vi "STM Multi-Client - Command Server.vi"() -> ()   [LabVIEW 2016]
uses:
  <vilib>/NI/STM/Connection Manager/TCP/TCP Connection Method.ctl
  <vilib>/NI/STM/SubVIs/MetaDataElement.ctl
  <vilib>/Platform/TimedLoop/XDataNode/timing_clust.ctl
  <vilib>/Platform/TimedLoop/XDataNode/nitl_modes.ctl
  <vilib>/Platform/TimedLoop/XDataNode/wakeup.ctl
  <vilib>/NI/STM/TCP/Write Meta Data (TCP Ref).vi
  <vilib>/NI/STM/TCP/Read Message (TCP).vi
  <vilib>/NI/STM/TCP/Write Message (TCP).vi
  <vilib>/NI/STM/TCP/Write Meta Data (TCP Clst).vi
  <vilib>/Platform/TimedLoop/XDataNode/XDataNode.xnode
  <vilib>/Platform/TimedLoop/XDataNode/XDNodeRunTimeDep.lvlib
  <vilib>/NI/STM/NI STM.lvlib
panel:
  in  "Stop non-critical loops":bool
  out "error out":errorcluster
  out "Number of \nConnections":i32
  # "Overview: Demonstrate the use of the STM library to implement a Single Server Multi Client application design. \nRequirements: LabVIEW Full Development System, STM Library version 3.x or later\nInstructions: \n1. Run the STM Multi-Client - Server VI\n2. Set the Target IP Address in the STM Multi-Client - Client VI to match the IP address of the server\n3. Run the STM Multi-Client - Client VI\n4. Change the Channel to choose between four different waveform"
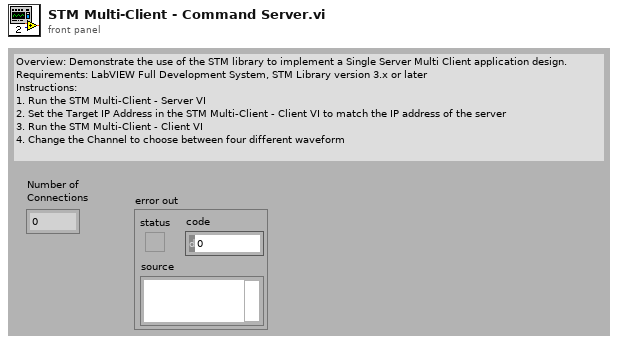
[diagram p1: front panel]
types:
  T1 = typedef "NI STM.lvlib/TCP Connection Method.ctl" = enum16{"Initialize", "Add Connection", "Set Properties", "Get Connection(s)", "Remove Connection", "Remove All Connections", "Get Connection Count"}
  T2 = typedef "NI STM.lvlib/MetaDataElement.ctl" = string
  T3 = typedef "FIFOs (STM Multi-Client).ctl" = cluster{"Data FIFO":refnum<queue>, "Stop FIFO":refnum<queue>}
  T4 = typedef "XDNodeRunTimeDep.lvlib/timing_clust.ctl" = cluster{"Expected End [f-1]":u64, "Actual End [f-1]":u64, "Finished Late? [f-1]":bool, "Expected End [i-1]":u64, "Actual End [i-1]":u64, "Finished Late? [i-1]":bool, "Expected Start [i]":u64, "Actual Start [i]":u64, "Expected Start [f]":u64, "Actual Start [f]":u64, "Source Name":string, "Structure Name":string, "Period":i64, "Deadline":i64, "Offset":i64, "Start":i64, "Priority":i32, "Timeout":i32, "Mode":T5, "Wakeup Reason":T6, "Error":errorcluster, "Source Type":string, "Secondary Source Type":string, "Global End Time":u64, "Global Start Time":u64, "Frame Duration":u64, "Iteration Duration":u64, "Assigned CPU":i32, "I/O Scan Engine Mode":u32}
  T5 = typedef "XDNodeRunTimeDep.lvlib/nitl_modes.ctl" = enum32{"No Change", "Process missed periods, maintain original phase", "Discard missed periods, maintain original phase", "Process missed periods, ignore original phase", "Discard missed periods, ignore original phase"}
  T6 = typedef "XDNodeRunTimeDep.lvlib/wakeup.ctl" = enum32{"Normal", "Aborted", "Asynchronous wakeup", "Timing source error", "Timed loop error", "Timeout"}
  T7 = typedef "NI STM.lvlib/TCP Connection Info.ctl" = cluster{"connection ID":refnum<k5>, "meta data":T2[]}
  T8 = typedef "NI STM.lvlib/TCP Connection Properties.ctl" = cluster{"Name":string, "Address":string, "Custom":string}
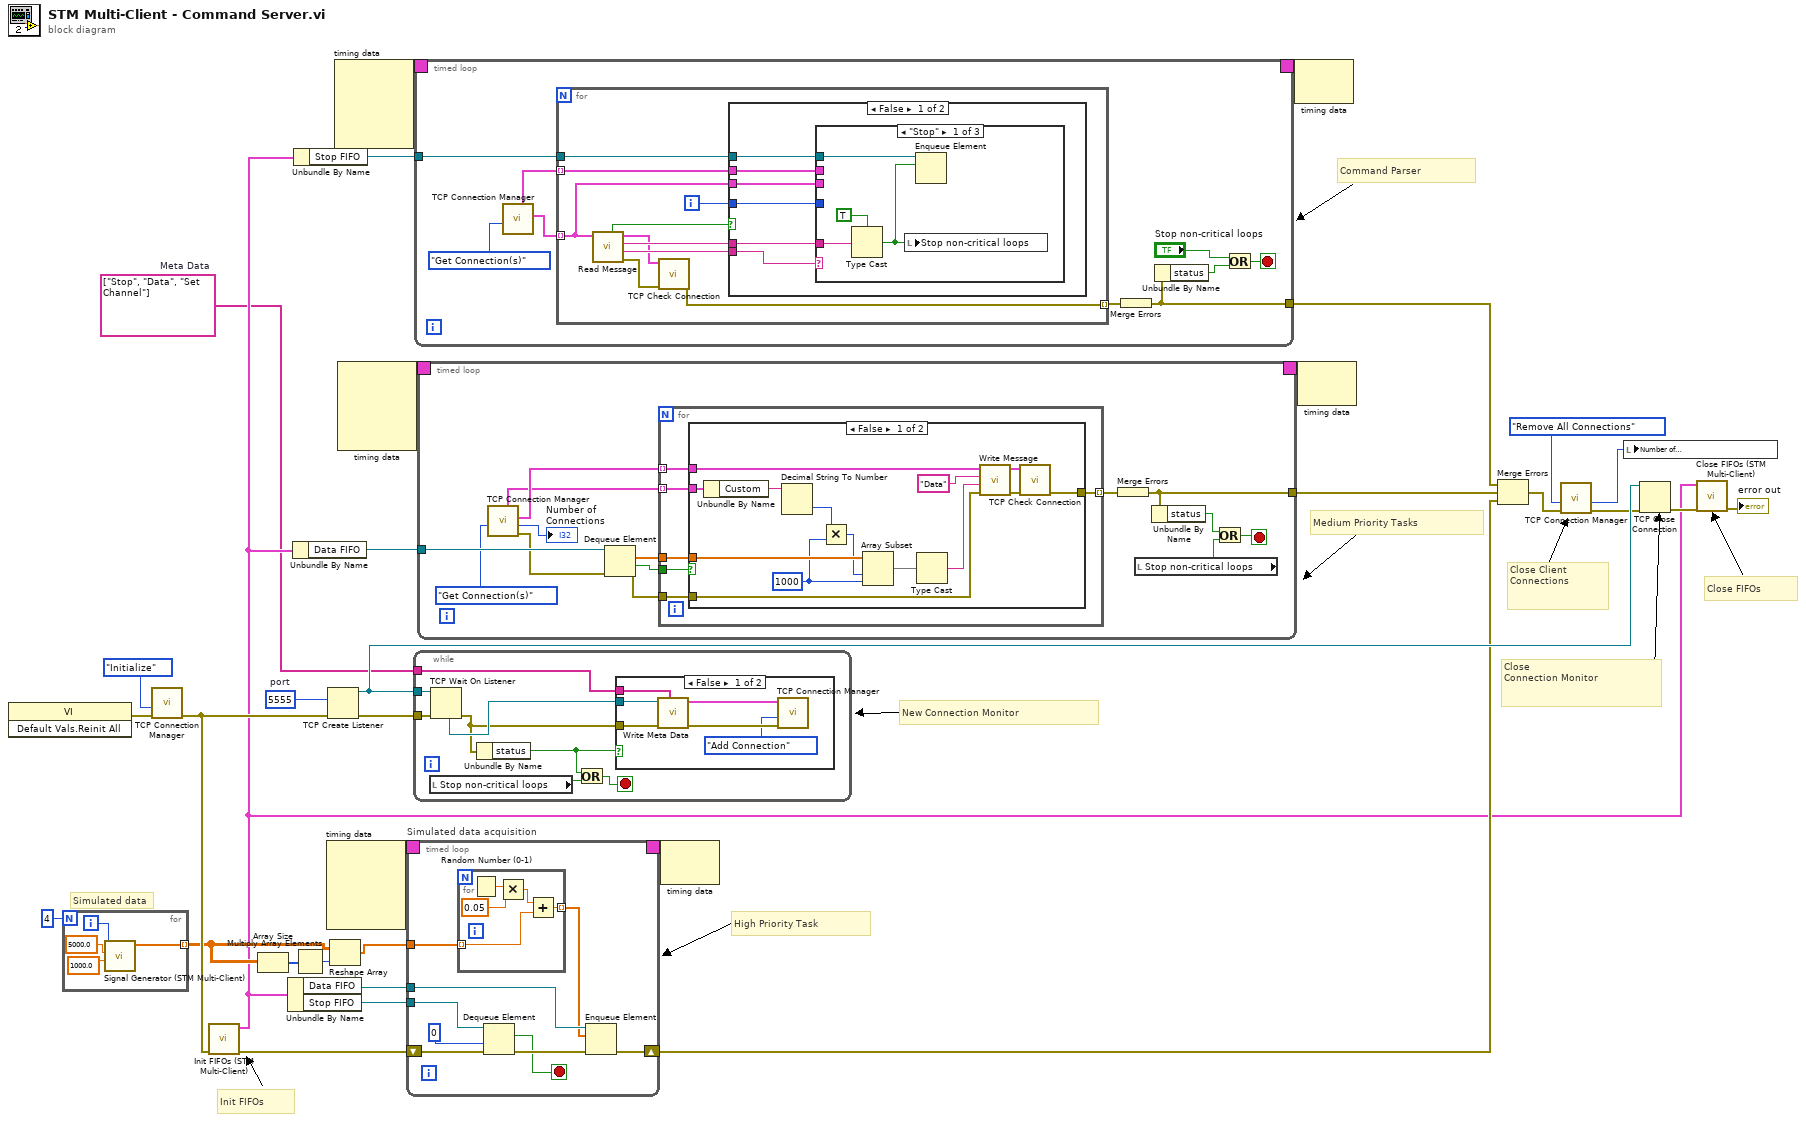
[diagram p0: block diagram]
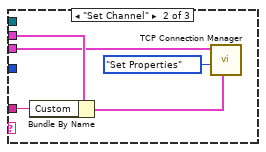
[diagram p3: hidden frame]
diagram:
  w2 = T2[] ["Stop", "Data", "Set Channel"]  # Meta Data
  w30 = u16 5555  # port
  # "Command Parser"
  # "Medium Priority Tasks"
  # "Close \nConnection Monitor"
  # "Init FIFOs"
  # "Simulated data"
  # "New Connection Monitor"
  # "Close Client\nConnections"
  # "Close FIFOs"
  # "High Priority Task"
  n1 = invoke class="VI" method="Default Vals.Reinit All"() -> (error out=w7:errorcluster)  [unwired: 3 in, 2 out]
  n2 = for {
    N: 4 -> [_]
    tunnel: [w36] -> w16 mode=indexing
    i -> [w37]
    n3 = call "Signal Generator (STM Multi-Client).vi"("#Samples"=1000.0, "frequency"=5000.0, "Signal Type"=w37) -> ("Data"=w36:dbl[])  [unwired: 7 in, 1 out]
  }
  n4 = call <vilib>:"TCP Connection Manager.vi"("error in"=w7, "method"=TCP_Connection_Method."Initialize") -> ("error out"=w28:errorcluster)  [unwired: 4 in, 5 out]
  n5 = call "Init FIFOs (STM Multi-Client).vi"("error in (no error)"=w28) -> ("error out"=w10:errorcluster, "FIFOs out"=w8:T3)  [unwired: 9 in]
  n6 = Array Size(array=w16) -> (size(s)=w15:i32[])
  n7 = Unbundle By Name(w8) -> ("Data FIFO"=w11:refnum<queue>, "Stop FIFO"=w12:refnum<queue>)
  n8 = Unbundle By Name(w8) -> ("Data FIFO"=w26:refnum<queue>)
  n9 = Unbundle By Name(w8) -> ("Stop FIFO"=w25:refnum<queue>)
  n10 = Multiply Array Elements(1:w15) -> (0:w14:i32)
  n11 = node-c288() -> (w19:T4)  [unwired: 4 in]
  n12 = TCP Create Listener(8:w28, 10:w30) -> (0:w31:errorcluster, 3:w29:refnum<k5>)  [unwired: 3 in, 1 out]
  n13 = Reshape Array(w16, w14) -> (w13:dbl[])
  n14 = node-c288() -> (w23:T4)  [unwired: 4 in]
  n15 = node-c288() -> (w21:T4)  [unwired: 4 in]
  n16 = timed-loop "Simulated data acquisition" {
    tunnel: w13 -> [w43]
    tunnel: w12 -> [w42]
    tunnel: w11 -> [w40]
    timing: w19 -> [_]
    timing-out: [_] -> w18
    shift-right: [w44] -> w9
    shift-left: w10 -> [w46]
    stop <- w41 stop-if-true
    n17 = for {
      tunnel: w43 -> [w48] mode=indexing
      tunnel: [w47] -> w39 mode=indexing
      n18 = Random Number (0-1)() -> (number: 0 to 1=w51:dbl)
      n19 = Multiply(x=w51, y=0.05) -> (x*y=w49:dbl)
      n20 = Add(x=w49, y=w48) -> (x+y=w47:dbl)
    }
    n21 = Dequeue Element(queue=w42, timeout in ms (-1)=0, error in (no error)=w46) -> (element=w41:bool, error out=w45:errorcluster)  [unwired: 2 out]
    n22 = Enqueue Element(queue=w40, element=w39, error in (no error)=w45) -> (error out=w44:errorcluster)  [unwired: 1 in, 2 out]
  }
  n23 = while "Listen loop.  Append new connections to a synchronized queue." {
    tunnel: w29 -> [w60]
    tunnel: w31 -> [w61]
    tunnel: w2 -> [w57]
    stop <- w55 stop-if-true
    n24 = local read "Stop non-critical loops"() -> (w54:bool)
    n25 = TCP Wait On Listener(8:w61, 11:w60) -> (0:w56:errorcluster, 4:w59:refnum<k5>)  [unwired: 2 in, 3 out]
    n26 = Unbundle By Name(w56) -> ("status"=w58:bool)
    n27 = Or(x=w58, y=w54) -> (x .or. y?=w55:bool)
    n28 = case shown="False" w58 {
      tunnel: w59 -> [w67 _]
      tunnel: w57 -> [w62 _]
      tunnel: w56 -> [w65 _]
      frame False {
        n29 = call-poly <vilib>:"Write Meta Data.vi"("meta data"=w62, "error in"=w65, "connection ID"=w67) -> ("error out"=w66:errorcluster, "connection info out"=w63:T7)  [unwired: 7 in]
        n30 = call <vilib>:"TCP Connection Manager.vi"("error in"=w66, "method"=TCP_Connection_Method."Add Connection", "connection in"=w63) -> ()  [unwired: 3 in, 6 out]
      }
      frame True {
      }
    }
  }
  n31 = timed-loop {
    tunnel: [w73] -> w32
    tunnel: w25 -> [w71]
    timing: w23 -> [_]
    timing-out: [_] -> w22
    stop <- w76 stop-if-true
    n32 = call <vilib>:"TCP Connection Manager.vi"("method"=TCP_Connection_Method."Get Connection(s)") -> ("all connections"=w72:T7[], "all properties"=w70:T8[])  [unwired: 5 in, 4 out]
    n33 = for {
      tunnel: [w82] -> w74 mode=indexing
      tunnel: w72 -> [w78] mode=indexing
      tunnel: w71 -> [w81]
      tunnel: w70 -> [w79] mode=indexing
      i -> [w80]
      n34 = call-poly <vilib>:"Read Message.vi"("connection info in"=w78) -> ("error out"=w83:errorcluster, "name"=w86:T2, "data string"=w85:string, "connection info out"=w77:T7, "timed out?"=w84:bool)  [unwired: 5 in, 1 out]
      n35 = call <vilib>:"TCP Check Connection.vi"("error in"=w83, "connection in"=w77) -> ("error out"=w82:errorcluster)  [unwired: 7 in, 2 out]
      n36 = case shown="False" w84 {
        tunnel: w86 -> [w87 _]
        tunnel: w85 -> [w92 _]
        tunnel: w81 -> [w91 _]
        tunnel: w78 -> [w90 _]
        tunnel: w80 -> [w89 _]
        tunnel: w79 -> [w88 _]
        frame False {
          n37 = case shown="\"Stop\"" w87 {
            tunnel: w92 -> [w96 w99 _]
            tunnel: w91 -> [w93 _ _]
            tunnel: w90 -> [_ w98 _]
            tunnel: w89 -> [_ _ _]
            tunnel: w88 -> [_ w101 _]
            frame "Stop" {
              n38 = Type Cast(type=TRUE, x=w96) -> (*(type *) &x=w94:bool)
              n39 = local write "Stop non-critical loops"(w94) -> ()
              n40 = Enqueue Element(queue=w93, element=w94) -> ()  [unwired: 2 in, 3 out]
            }
            frame "Set Channel" {
              n41 = Bundle By Name(cluster=w101, "Custom"=w99) -> (w100:T8)
              n42 = call <vilib>:"TCP Connection Manager.vi"("properties in"=w100, "method"=TCP_Connection_Method."Set Properties", "connection in"=w98) -> ()  [unwired: 3 in, 6 out]
            }
            frame Default {
            }
          }
        }
        frame True {
        }
      }
    }
    n43 = Merge Errors(w74) -> (w73:errorcluster)
    n44 = Unbundle By Name(w73) -> ("status"=w75:bool)
    n45 = Or(x="Stop non-critical loops", y=w75) -> (x .or. y?=w76:bool)
  }
  n46 = timed-loop {
    tunnel: [w111] -> w33
    tunnel: w26 -> [w109]
    timing: w21 -> [_]
    timing-out: [_] -> w20
    stop <- w117 stop-if-true
    n47 = call <vilib>:"TCP Connection Manager.vi"("method"=TCP_Connection_Method."Get Connection(s)") -> ("error out"=w104:errorcluster, "number of connections"=→"Number of \nConnections":i32, "all connections"=w114:T7[], "all properties"=w110:T8[])  [unwired: 5 in, 2 out]
    n48 = Dequeue Element(queue=w109, error in (no error)=w104) -> (element=w108:dbl[], timed out?=w107:bool, error out=w105:errorcluster)  [unwired: 1 in, 1 out]
    n49 = for {
      tunnel: [w122] -> w113 mode=indexing
      tunnel: w114 -> [w123] mode=indexing
      tunnel: w110 -> [w121] mode=indexing
      tunnel: w108 -> [w120]
      tunnel: w107 -> [w119]
      tunnel: w105 -> [w118]
      n50 = case shown="False" w119 {
        tunnel: w123 -> [w126 _]
        tunnel: [w135 _] -> w122
        tunnel: w120 -> [w133 _]
        tunnel: w121 -> [w132 _]
        tunnel: w118 -> [w124 _]
        frame False {
          w131 = 1000 ("length")
          n51 = Unbundle By Name(w132) -> ("Custom"=w130:string)
          n52 = Decimal String To Number(string=w130) -> (number=w127:i32)  [unwired: 2 in, 1 out]
          n53 = Multiply(x=w127, y=w131) -> (x*y=w129:i32)
          n54 = Array Subset(array=w133, index=w129, length=w131) -> (w128:dbl[])
          n55 = Type Cast(x=w128) -> (*(type *) &x=w134:string)  [unwired: 1 in]
          n56 = call-poly <vilib>:"Write Message.vi"("error in"=w124, "data"=w134, "name"="Data" ("Name"), "connection info in"=w126) -> ("error out"=w136:errorcluster, "connection info out"=w125:T7)  [unwired: 6 in]
          n57 = call <vilib>:"TCP Check Connection.vi"("error in"=w136, "connection in"=w125) -> ("error out"=w135:errorcluster)  [unwired: 7 in, 2 out]
        }
        frame True {
        }
      }
    }
    n58 = Merge Errors(w113) -> (w111:errorcluster)
    n59 = local read "Stop non-critical loops"() -> (w115:bool)
    n60 = Unbundle By Name(w111) -> ("status"=w116:bool)
    n61 = Or(x=w116, y=w115) -> (x .or. y?=w117:bool)
  }
  n62 = node-c288(w18) -> ()  [unwired: 1 out]
  n63 = node-c288(w22) -> ()  [unwired: 1 out]
  n64 = node-c288(w20) -> ()  [unwired: 1 out]
  n65 = Merge Errors(w32, w33, w9) -> (w6:errorcluster)
  n66 = call <vilib>:"TCP Connection Manager.vi"("error in"=w6, "method"=TCP_Connection_Method."Remove All Connections") -> ("error out"=w5:errorcluster, "number of connections"=w4:i32)  [unwired: 4 in, 4 out]
  n67 = local write "Number of \nConnections"(w4) -> ()
  n68 = TCP Close Connection(connection ID=w29, error in (no error)=w5) -> (error out=w27:errorcluster)  [unwired: 1 in, 1 out]
  n69 = call "Close FIFOs (STM Multi-Client).vi"("error in (no error)"=w27, "FIFOs In"=w8) -> ("error out"=→"error out":errorcluster)  [unwired: 9 in]
